vi "checkTolerance.vi"(9 "Tolerance":dbl[unit], 10 "Expected Value":dbl[unit], 11 "Average":dbl) -> (3 "Boolean":bool)   [LabVIEW 2015]
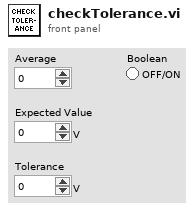
[diagram p1: front panel]
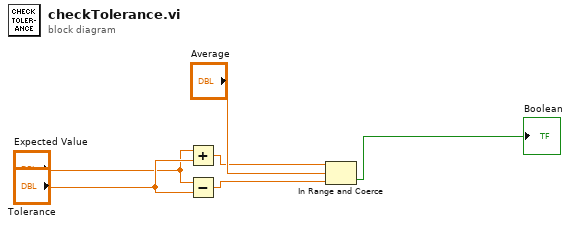
[diagram p0: block diagram]
diagram:
  n1 = Add(x="Expected Value", y="Tolerance") -> (x+y=w3:dbl[unit])
  n2 = Subtract(x="Expected Value", y="Tolerance") -> (x-y=w4:dbl[unit])
  n3 = In Range and Coerce(upper limit=w3, x="Average", lower limit=w4) -> (In Range?=→"Boolean":bool)  [unwired: 1 out]
